vi "InitTH260_UIThread.vi"(8 "error in (no error)":errorcluster, 9 "MeasMode":T3 items=["Histo"=0, "T2"=2, "T3"=3, "Conti"=8], 10 "TimingMode":T1 items=["Hires", "Lowres"], 11 "Library Version":string="3.1") -> (0 "error out":errorcluster, 2 "Init Info":T2, 3 "DevIdx":i32)   [LabVIEW 2010]
uses:
  TH260_InitInfo.ctl
  TH260_MeasMode.ctl
  TH260_TimingMode.ctl
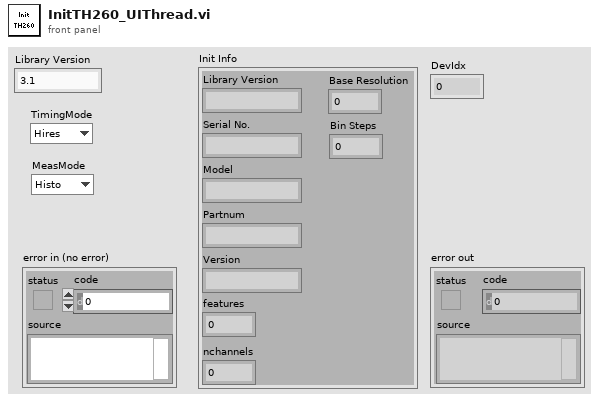
[diagram p1: front panel]
types:
  T1 = typedef "TH260_TimingMode.ctl" = i32
  T2 = typedef "TH260_InitInfo.ctl" = cluster{"Library Version":string, "Serial No.":string, "Model":string, "Partnum":string, "Version":string, "features":i32, "nchannels":i32, "Base Resolution":dbl, "Bin Steps":i32}
  T3 = typedef "TH260_MeasMode.ctl" = i32
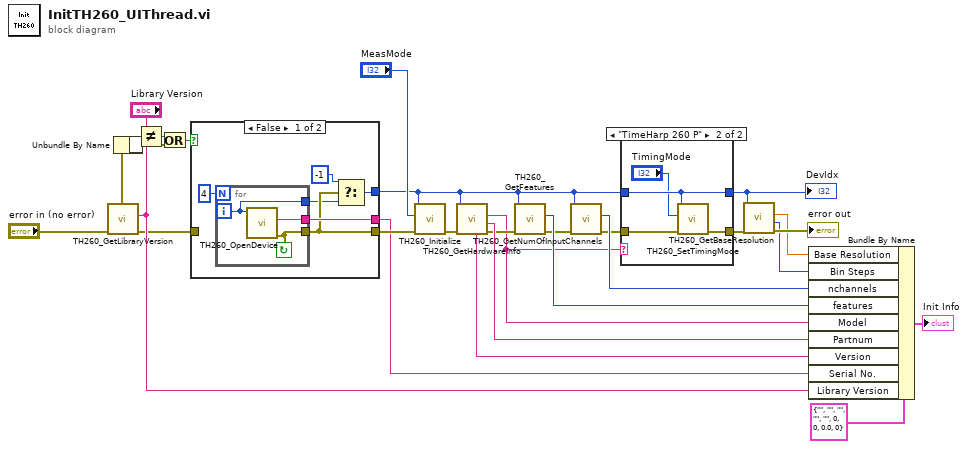
[diagram p0: block diagram]
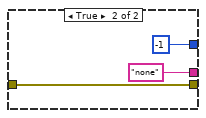
[diagram p3: hidden frame]
diagram:
  n1 = call "TH260_GetLibraryVersion.vi"("error in (no error)"="error in (no error)") -> ("error out"=w8:errorcluster, "Version"=w16:string)  [unwired: 8 in, 1 out]
  n2 = Not Equal?(x="Library Version", y=w16) -> (x != y?=w26:bool)
  n3 = Or(x=w26) -> (y=w1:errorcluster, x .or. y?=w25:bool)
  n4 = Unbundle By Name(w8, w1) -> ()
  n5 = case shown="False" w25 {
    tunnel: [w29 -1 ("return type")] -> w5
    tunnel: [w32 "none" ("serial")] -> w18
    tunnel: [w31 w37] -> w24
    tunnel: w8 -> [_ w37]
    frame False {
      n6 = for {
        N: 4 -> [_]
        tunnel: [w35] -> w31
        tunnel: [w34] -> w32
        tunnel: [w36] -> w30
        i -> [w36]
        stop <- w35 continue-if-true
        n7 = call "TH260_OpenDevice.vi"("devidx"=w36) -> ("error out"=w35:errorcluster, "serial"=w34:string)  [unwired: 8 in, 1 out]
      }
      n8 = Select(t=-1, s=w31, f=w30) -> (s? t:f=w29:i32)
    }
    frame True {
    }
  }
  n9 = call "TH260_Initialize.vi"("error in (no error)"=w24, "mode"="MeasMode", "devidx"=w5) -> ("error out"=w22:errorcluster)  [unwired: 7 in, 1 out]
  n10 = call "TH260_GetHardwareInfo.vi"("error in (no error)"=w22, "devidx"=w5) -> ("error out"=w14:errorcluster, "Partnum"=w21:string, "Model"=w6:string, "Version"=w20:string)  [unwired: 5 in, 1 out]
  n11 = call "TH260_GetFeatures.vi"("error in (no error)"=w14, "devidx"=w5) -> ("error out"=w7:errorcluster, "features"=w19:i32)  [unwired: 7 in, 1 out]
  n12 = call "TH260_GetNumOfInputChannels.vi"("error in (no error)"=w7, "devidx"=w5) -> ("error out"=w4:errorcluster, "nchannels"=w13:i32)  [unwired: 7 in, 1 out]
  n13 = case shown="\"TimeHarp 260 P\"" w6 {
    tunnel: w5 -> [w40 w43]
    tunnel: w4 -> [w41 w45]
    tunnel: [w41 w44] -> w3
    tunnel: [w40 w43] -> w2
    frame Default {
    }
    frame "TimeHarp 260 P" {
      n14 = call "TH260_SetTimingMode.vi"("error in (no error)"=w45, "mode"="TimingMode", "devidx"=w43) -> ("error out"=w44:errorcluster)  [unwired: 7 in, 1 out]
    }
  }
  "DevIdx" <- w2
  n15 = call "TH260_GetBaseResolution.vi"("error in (no error)"=w3, "devidx"=w2) -> ("error out"=→"error out":errorcluster, "binsteps"=w11:i32, "resolution"=w10:dbl)  [unwired: 6 in, 1 out]
  n16 = Bundle By Name(cluster=T2 {"Library Version"="", "Serial No."="", "Model"="", "Partnum"="", "Version"="", "features"=0, "nchannels"=0, "Base Resolution"=0.0, "Bin Steps"=0} ("Init"), "Base Resolution"=w10, "Bin Steps"=w11, "nchannels"=w13, "features"=w19, "Model"=w6, "Partnum"=w21, "Version"=w20, "Serial No."=w18, "Library Version"=w16) -> (→"Init Info":T2)
